vi "Write TDATA Core.vi"(10 "raw data":bool[](array[boolean]), 11 "niInstr AXI4-Stream Writer FXP64x2 v1 FPGA in":refnum<class "niInstr AXI4-Stream Writer FXP64x2 v1 FPGA.lvclass">) -> (3 "niInstr AXI4-Stream Writer FXP64x2 v1 FPGA out":refnum<class "niInstr AXI4-Stream Writer FXP64x2 v1 FPGA.lvclass">)   [LabVIEW 2015, in "niInstr AXI4-Stream Writer FXP64x2 v1 FPGA.lvclass"]
uses:
  <instrlib>/_niInstr/CLIP Adapters/v1/FPGA/AXI4-Stream/Writer FXP64x2/niInstr AXI4-Stream Writer FXP64x2 v1 FPGA.lvclass
  <instrlib>/_niInstr/CLIP Adapters/v1/FPGA/AXI4-Stream/Writer FXP64x2/niInstr AXI4-Stream Writer FXP64x2 v1 FPGA.lvclass/niInstr AXI4-Stream Writer FXP64x2 v1 FPGA.ctl
  <vilib>/rvi/eio/common/nirviEmuTemplateMethod_errors.vi
  <instrlib>/_niInstr/Data Formatting/v1/FPGA/Private/Convert/Boolean Array to U64 Array.vi
  <vilib>/eio/EIONode/EIONode.xnode
  <instrlib>/_niInstr/Data Formatting/v1/FPGA/niInstr Data Formatting v1 FPGA.lvlib
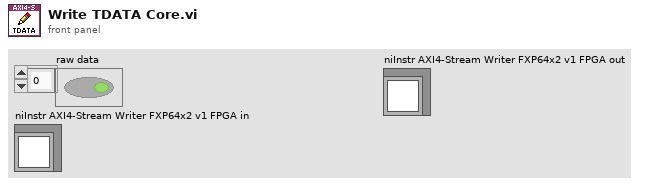
[diagram p1: front panel]
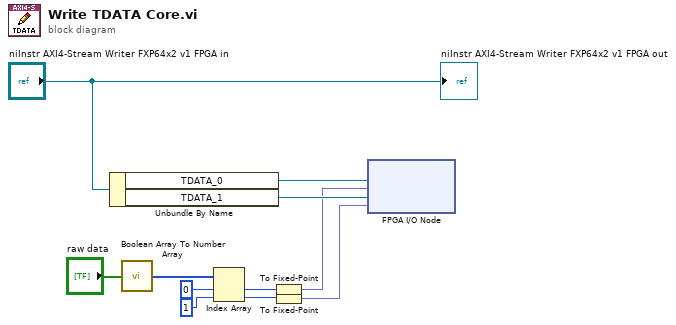
[diagram p0: block diagram]
diagram:
  n1 = Unbundle By Name("niInstr AXI4-Stream Writer FXP64x2 v1 FPGA in") -> ("TDATA_0"=w10:refnum<k21>, "TDATA_1"=w9:refnum<k21>)
  n2 = call-poly <instrlib>:"Boolean Array To Number Array.vi"("data in"="raw data") -> ("data out"=w5:u64[])  [unwired: 14 in]
  n3 = Index Array(array=w5, index #1=0 ("index"), index #2=1 ("index")) -> (element #1=w4:u64, element #2=w2:u64)
  n4 = To Fixed-Point(number=w4) -> (fixed-point=w3:fxp<+,64,64>)  [unwired: 1 in]
  n5 = To Fixed-Point(number=w2) -> (fixed-point=w1:fxp<+,64,64>)  [unwired: 1 in]
  n6 = xnode "FPGA I/O Node"("I/O Item"=w3, "FPGA I/O In"=w10, "I/O Item"=w1, "FPGA I/O In"=w9) -> ()  [unwired: 2 out]
  "niInstr AXI4-Stream Writer FXP64x2 v1 FPGA out" <- "niInstr AXI4-Stream Writer FXP64x2 v1 FPGA in"
